vi "Begin.vi"() -> (0 "error out":errorcluster)   [LabVIEW 2013]
doc: "Called before other user functions, this VI is expected to open initial I/O refnums, load in file data, and do all program initialization. Notice that the <B>error out</B> terminal is simply used for data flow. Wiring it to other structures or subVIs ensures that this VI runs first."
uses:
  Robot Global Data.vi
  <vilib>/Rock Robotics/WPI/DriverStation/WPI_DriverStationRobotMode2.ctl
  DBNameEnum.ctl
  <vilib>/Rock Robotics/WPI/Solenoid/WPI_SolenoidOpenSingle.vi
  ShooterOperation.ctl
  <vilib>/Rock Robotics/WPI/SafetyOutput/WPI_SafetyOutputConfigMenu.ctl
  <vilib>/Rock Robotics/WPI/RobotDrive/WPI_RobotDriveOpen2MotorWithTalon.vi
  TankDriveEnum.ctl
  <vilib>/Rock Robotics/WPI/Joystick/WPI_JoystickDeviceEnum.ctl
  RefnameEnum.ctl
  PnuematicMode.ctl
  RollerStates.ctl
panel:
  in  "Version":string="TF 2.1.5"
  # "SET AS DEFAULT"
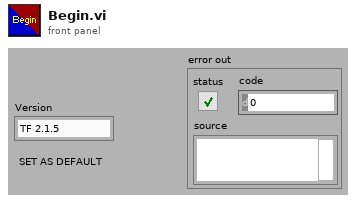
[diagram p1: front panel]
types:
  T1 = typedef "RefnameEnum.ctl" = enum16{"TankDrive", "Controller1", "Controller2", "SonicShifter", "Compressor"}
  T2 = typedef "RollerStates.ctl" = enum16{"Init", "SetState", "Disable"}
  T3 = typedef "PnuematicMode.ctl" = enum16{"Init", "SetState", "Disable"}
  T4 = typedef "WPI_JoystickDeviceEnum.ctl" = enum16{"USB 1", "USB 2", "USB 3", "USB 4", "Kinect 1", "Kinect 2"}
  T5 = typedef "TankDriveEnum.ctl" = enum16{"Init", "LinearDrive", "SetValue", "Disable"}
  T6 = typedef "WPI_SafetyOutputConfigMenu.ctl" = enum16{"Enable", "Disable"}
  T7 = typedef "ShooterOperation.ctl" = enum16{"Init", "ExtendKicker", "RetractKicker", "Shoot", "RetractShooter"}
  T8 = typedef "DBNameEnum.ctl" = enum16{"Version"}
  T9 = typedef "WPI_DriverStationRobotMode2.ctl" = enum16{"Autonomous Disabled", "Autonomous Enabled", "Teleop Disabled", "Teleop Enabled", "Timeout", "Finish", "Test Disabled", "Test Enabled"}
  T10 = typedef "WPI_JoystickDevRef.ctl" = cluster{"Device":T4}
  T11 = typedef "WPI_RobotDriveDevRef.ctl" = cluster{"DevStatus":errorcluster, "Motors[]":T12[], "Square Inputs":bool, "Max Output":dbl, "Isochronous":bool}
  T12 = typedef "WPI_MotorControlDeviceRef.ctl" = cluster{"DeviceStatus":errorcluster, "Type":enum16{"PWM", "CAN"}, "PWM":cluster{"Digital Module":T13, "PWM Channel":T14, "DeadBand":T15}, "CAN":cluster{"Device Number":u8, "Control Mode":T16, "Semaphore":T17, "Max Vout":dbl}, "Invert":bool, "TransformRef":T18, "InvTransformRef":T18}
  T13 = typedef "FPGA_TypedefDigitalModule.ctl" = enum16{"Digital Module 1", "Digital Module 2"}
  T14 = typedef "FPGA_DIOPWMChannel.ctl" = enum8{"PWM 1", "PWM 2", "PWM 3", "PWM 4", "PWM 5", "PWM 6", "PWM 7", "PWM 8", "PWM 9", "PWM 10", "Invalid"}
  T15 = typedef "WPI_PWMDeadband.ctl" = cluster{"Name":string, "maxPositivePwm":i32, "minPositivePwm":i32, "centerPwm":i32, "maxNegativePwm":i32, "minNegativePwm":i32, "angularRange":u16}
  T16 = typedef "WPI_CANJaguar_ControlMode.ctl" = enum8{"Percent VBus", "Current", "Speed", "Position", "Voltage"}
  T17 = typedef "Semaphore RefNum" = refnum<k1>
  T18 = typedef "WPI_PWMTransform_ConPane.ctl" = refnum<vi>
  T19 = typedef "WPI_SolenoidDevRef.ctl" = cluster{"DevStatus":errorcluster, "Solenoid Module":T20, "Forward Solenoid Channel":T21, "Reverse Solenoid Channel":T21}
  T20 = typedef "FPGA_TypedefSolenoidModule.ctl" = enum16{"Solenoid Module 1", "Solenoid Module 2"}
  T21 = typedef "WPI_SolenoidChannel.ctl" = enum8{"Solenoid 1", "Solenoid 2", "Solenoid 3", "Solenoid 4", "Solenoid 5", "Solenoid 6", "Solenoid 7", "Solenoid 8", "Invalid"}
  T22 = typedef "WPI_CompressorDevRef.ctl" = cluster{"DevStatus":errorcluster, "DigitalInputDevRef":T23, "RelayDevRef":T25}
  T23 = typedef "WPI_DigitalInputDevRef.ctl" = cluster{"DevStatus":errorcluster, "DIO Channel":T24, "Digital Module":T13}
  T24 = typedef "FPGA_DIOChannel.ctl" = enum8{"DIO 1", "DIO 2", "DIO 3", "DIO 4", "DIO 5", "DIO 6", "DIO 7", "DIO 8", "DIO 9", "DIO 10", "DIO 11", "DIO 12", "DIO 13", "DIO 14", "Invalid"}
  T25 = typedef "WPI_RelayDevRef.ctl" = cluster{"DevStatus":errorcluster, "Relay Channel":T26, "Digital Module":T13, "Relay Direction":T27}
  T26 = typedef "FPGA_DIORelayChannel.ctl" = enum8{"Relay 1", "Relay 2", "Relay 3", "Relay 4", "Relay 5", "Relay 6", "Relay 7", "Relay 8", "Invalid"}
  T27 = typedef "WPI_RelayDirection.ctl" = enum16{"Both directions", "Forward only", "Reverse only"}
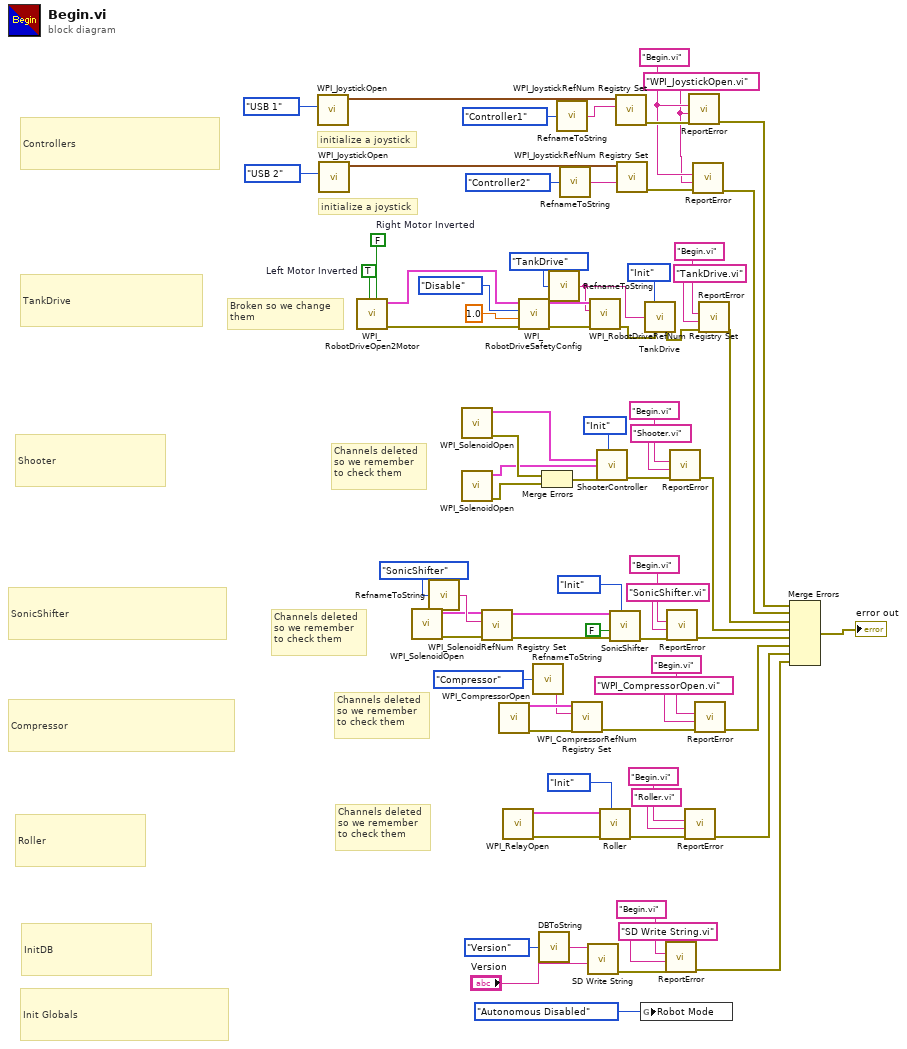
[diagram p0: block diagram]
diagram:
  w45 = "WPI_JoystickOpen.vi" ("Causing VI")
  w46 = "Begin.vi" ("Calling VI")
  w62 = FALSE  # Right Motor Inverted
  w61 = TRUE  # Left Motor Inverted
  # "Channels deleted\nso we remember\nto check them"
  # "Compressor"
  # "Roller"
  # "Channels deleted\nso we remember\nto check them"
  # "Channels deleted\nso we remember\nto check them"
  # "SonicShifter"
  # "Controllers"
  # "initialize a joystick"
  # "initialize a joystick"
  # "TankDrive"
  # "Broken so we change\nthem"
  # "Init Globals"
  # "InitDB"
  # "Shooter"
  # "Channels deleted\nso we remember\nto check them"
  n1 = call <vilib>:"WPI_JoystickOpen.vi"("JoystickDevice"=WPI_JoystickDeviceEnum."USB 1") -> ("JoystickDevRef"=w56:T10)  [unwired: 10 in]
  n2 = call <vilib>:"WPI_JoystickOpen.vi"("JoystickDevice"=WPI_JoystickDeviceEnum."USB 2") -> ("JoystickDevRef"=w53:T10)  [unwired: 10 in]
  n3 = call-poly <vilib>:"WPI_RobotDriveOpen2Motor.vi"("Right Motor Inverted"=w62, "Left Motor Inverted"=w61) -> ("error out"=w65:errorcluster, "RobotDriveDevRef"=w68:T11)  [unwired: 8 in]
  n4 = call-poly <vilib>:"WPI_SolenoidOpen.vi"() -> ("error out"=w35:errorcluster, "SolenoidDevRef"=w32:T19)  [unwired: 10 in]
  n5 = call "RefnameToString.vi"("Enum"=RefnameEnum."SonicShifter") -> ("Refname"=w33:string)
  n6 = call-poly <vilib>:"WPI_SolenoidOpen.vi"() -> ("error out"=w23:errorcluster, "SolenoidDevRef"=w21:T19)  [unwired: 10 in]
  n7 = call-poly <vilib>:"WPI_SolenoidOpen.vi"() -> ("error out"=w22:errorcluster, "SolenoidDevRef"=w20:T19)  [unwired: 10 in]
  n8 = call <vilib>:"WPI_SolenoidRefNum Registry Set.vi"("error in (no error)"=w35, "refnum name"=w33, "SolenoidDevRef"=w32) -> ("error out"=w31:errorcluster, "SolenoidDevRef"=w26:T19)  [unwired: 7 in]
  n9 = call <vilib>:"WPI_CompressorOpen.vi"() -> ("CompressorDevRef"=w8:T22, "error out"=w7:errorcluster)  [unwired: 5 in, 9 out]
  n10 = call <vilib>:"WPI_RelayOpen.vi"() -> ("error out"=w16:errorcluster, "RelayDevRef"=w14:T25)  [unwired: 10 in]
  n11 = call <vilib>:"WPI_RobotDriveSafetyConfig.vi"("error in (no error)"=w65, "timeout (s)"=1.0, "mode"=WPI_SafetyOutputConfigMenu."Disable", "RobotDriveDevRef"=w68) -> ("error out"=w66:errorcluster, "RobotDriveDevRef"=w67:T11)  [unwired: 6 in]
  n12 = call "RefnameToString.vi"("Enum"=RefnameEnum."Compressor") -> ("Refname"=w4:string)
  n13 = call "DBToString.vi"("Enum"=DBNameEnum."Version") -> ("Refname"=w73:string)
  n14 = Merge Errors(w23, w22) -> (w71:errorcluster)
  n15 = call "RefnameToString.vi"("Enum"=RefnameEnum."TankDrive") -> ("Refname"=w43:string)
  n16 = call "RefnameToString.vi"("Enum"=RefnameEnum."Controller1") -> ("Refname"=w41:string)
  n17 = call "RefnameToString.vi"("Enum"=RefnameEnum."Controller2") -> ("Refname"=w39:string)
  n18 = call <vilib>:"WPI_CompressorRefNum Registry Set.vi"("error in (no error)"=w7, "refnum name"=w4, "CompressorDevRef"=w8) -> ("error out"=w6:errorcluster)  [unwired: 7 in, 1 out]
  n19 = call <vilib>:"SD Write String.vi"("String"="Version", "Name"=w73) -> ("error out"=w36:errorcluster)  [unwired: 8 in, 1 out]
  n20 = call <vilib>:"WPI_RobotDriveRefNum Registry Set.vi"("error in (no error)"=w66, "refnum name"=w43, "RobotDriveDevRef"=w67) -> ("error out"=w59:errorcluster)  [unwired: 7 in, 1 out]
  n21 = call "ShooterController.vi"("Operation"=ShooterOperation."Init", "error in"=w71, "Kicker"=w20, "Shooter"=w21) -> ("error out"=w70:errorcluster)  [unwired: 7 in]
  n22 = call "Roller.vi"("Action"=RollerStates."Init" ("RollerState"), "error in"=w16, "RelayDevRef"=w14) -> ("error out"=w15:errorcluster)  [unwired: 8 in]
  n23 = call "SonicShifter.vi"("Mode"=PnuematicMode."Init", "error in (no error)"=w31, "Default Position"=FALSE, "SolenoidDevRef"=w26) -> ("error out"=w30:errorcluster)  [unwired: 7 in]
  n24 = call <vilib>:"WPI_JoystickRefNum Registry Set.vi"("refnum name"=w41, "JoystickDevRef"=w56) -> ("error out"=w47:errorcluster)  [unwired: 8 in, 1 out]
  n25 = call <vilib>:"WPI_JoystickRefNum Registry Set.vi"("refnum name"=w39, "JoystickDevRef"=w53) -> ("error out"=w50:errorcluster)  [unwired: 8 in, 1 out]
  n26 = global write "Robot Global Data.vi" "Robot Mode"(WPI_DriverStationRobotMode2."Autonomous Disabled" ("Robot Mode")) -> ()
  n27 = call "TankDrive.vi"("TankDriveEnum"=TankDriveEnum."Init", "MotorName"=w43, "error in (no error)"=w59) -> ("error out"=w58:errorcluster)  [unwired: 10 in, 2 out]
  n28 = call "ReportError.vi"("error in (no error)"=w36, "Causing VI"="SD Write String.vi", "Calling VI"="Begin.vi") -> ("error out"=w10:errorcluster)  [unwired: 8 in]
  n29 = call "ReportError.vi"("error in (no error)"=w30, "Causing VI"="SonicShifter.vi", "Calling VI"="Begin.vi") -> ("error out"=w29:errorcluster)  [unwired: 8 in]
  n30 = call "ReportError.vi"("error in (no error)"=w70, "Causing VI"="Shooter.vi" ("Calling VI"), "Calling VI"="Begin.vi") -> ("error out"=w19:errorcluster)  [unwired: 8 in]
  n31 = call "ReportError.vi"("error in (no error)"=w15, "Causing VI"="Roller.vi", "Calling VI"="Begin.vi") -> ("error out"=w9:errorcluster)  [unwired: 8 in]
  n32 = call "ReportError.vi"("error in (no error)"=w47, "Causing VI"=w45, "Calling VI"=w46) -> ("error out"=w48:errorcluster)  [unwired: 8 in]
  n33 = call "ReportError.vi"("error in (no error)"=w50, "Causing VI"=w45, "Calling VI"=w46) -> ("error out"=w49:errorcluster)  [unwired: 8 in]
  n34 = call "ReportError.vi"("error in (no error)"=w6, "Causing VI"="WPI_CompressorOpen.vi", "Calling VI"="Begin.vi") -> ("error out"=w3:errorcluster)  [unwired: 8 in]
  n35 = call "ReportError.vi"("error in (no error)"=w58, "Causing VI"="TankDrive.vi", "Calling VI"="Begin.vi") -> ("error out"=w57:errorcluster)  [unwired: 8 in]
  n36 = Merge Errors(w48, w49, w57, w19, w29, w3, w9, w10) -> (→"error out":errorcluster)
